vi "Connect to Data Server.vi"(8 "error in (no error)":errorcluster, 9 "timeout ms (60000)":i32=60000, 11 "server address":string) -> (0 "error out":errorcluster, 1 "timed out?":bool, 2 "framework configuration":T1, 3 "server ID":refnum<k5>)   [LabVIEW 2017, in "DSF Core.lvlib"]
uses:
  DSF Core.lvlib
  Typedefs/DSF Engine Framework Configuration.ctl
  Typedefs/DSF Engine Plugin Configuration.ctl
  Typedefs/DSF Timing Info.ctl
  Typedefs/DSF Engine Plugin Thread Configuration.ctl
  Typedefs/DSF Settings Info.ctl
  Typedefs/DSF Engine Transfer Group Configuration.ctl
  Typedefs/DSF Direction.ctl
  Typedefs/DSF Engine Transfer Configuration.ctl
  Typedefs/DSF Byte Order.ctl
  Typedefs/DSF Engine Channel Configuration.ctl
  Typedefs/DSF Data Type.ctl
  Typedefs/DSF Timeout Behavior.ctl
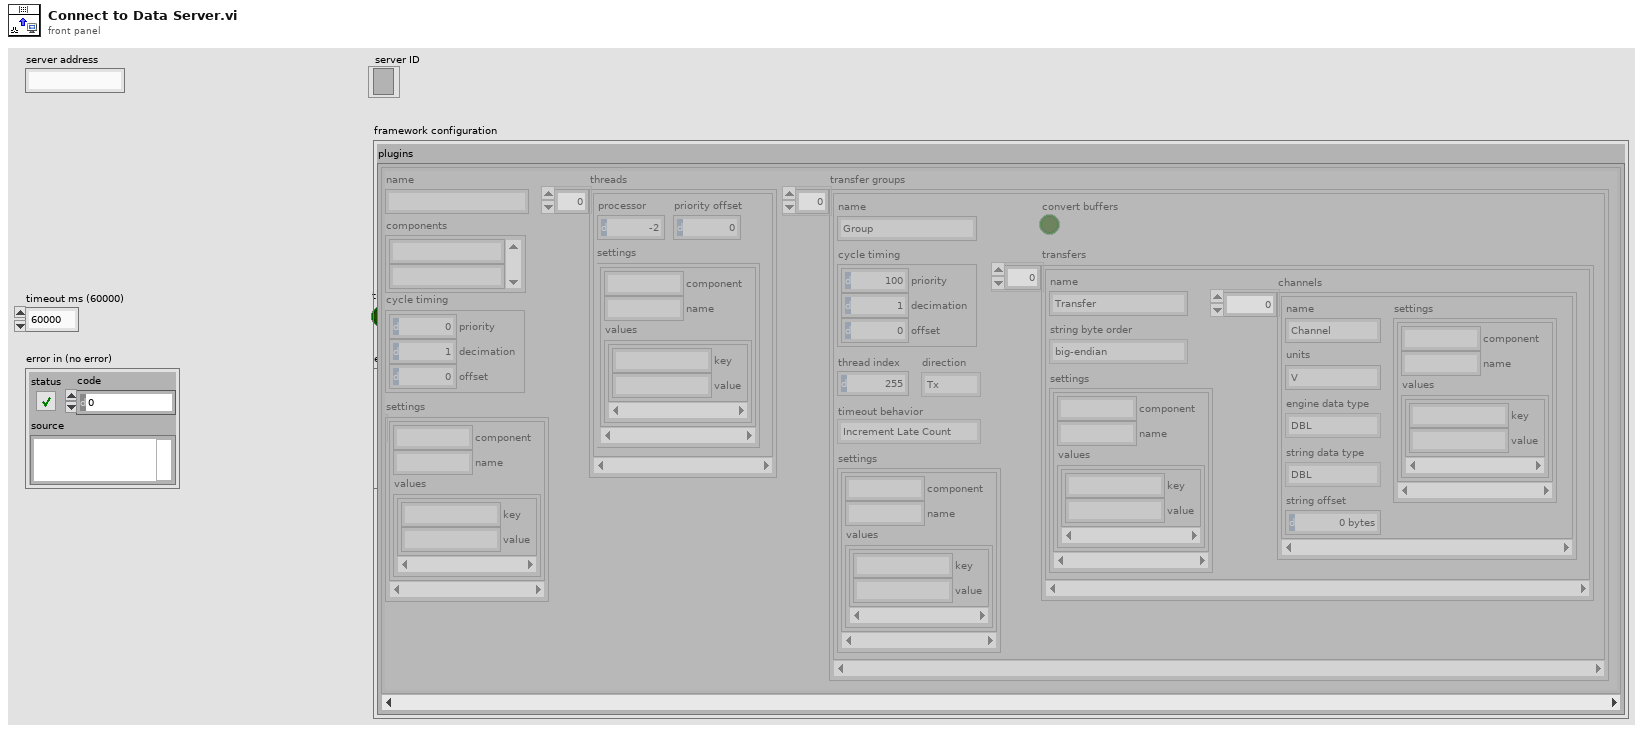
[diagram p1: front panel]
types:
  T1 = typedef "DSF Core.lvlib/DSF Engine Framework Configuration.ctl" = cluster{"plugins":T2[]}
  T2 = typedef "DSF Core.lvlib/DSF Engine Plugin Configuration.ctl" = cluster{"name":string, "components":string[], "cycle timing":T3, "threads":T4[], "transfer groups":T6[], "settings":T5}
  T3 = typedef "DSF Core.lvlib/DSF Timing Info.ctl" = cluster{"priority":u64, "decimation":u64, "offset":u64}
  T4 = typedef "DSF Core.lvlib/DSF Engine Plugin Thread Configuration.ctl" = cluster{"processor":i32, "priority offset":i16, "settings":T5}
  T5 = typedef "DSF Core.lvlib/DSF Settings Info.ctl" = cluster{"component":string, "name":string, "values":cluster{"key":string, "value":string}[]}[]
  T6 = typedef "DSF Core.lvlib/DSF Engine Transfer Group Configuration.ctl" = cluster{"name":string, "direction":T7, "cycle timing":T3, "thread index":u8, "settings":T5, "transfers":T8[], "timeout behavior":T12, "convert buffers":bool}
  T7 = typedef "DSF Core.lvlib/DSF Direction.ctl" = enum8{"Tx", "Rx"}
  T8 = typedef "DSF Core.lvlib/DSF Engine Transfer Configuration.ctl" = cluster{"name":string, "string byte order":T9, "settings":T5, "channels":T10[]}
  T9 = typedef "DSF Core.lvlib/DSF Byte Order.ctl" = enum8{"big-endian", "little-endian"}
  T10 = typedef "DSF Core.lvlib/DSF Engine Channel Configuration.ctl" = cluster{"string offset":u64, "name":string, "units":string, "engine data type":T11, "string data type":T11, "settings":T5}
  T11 = typedef "DSF Core.lvlib/DSF Data Type.ctl" = enum8{"Bool", "SGL", "DBL", "I8", "I16", "I32", "I64", "U8", "U16", "U32", "U64"}
  T12 = typedef "DSF Core.lvlib/DSF Timeout Behavior.ctl" = enum8{"Increment Late Count", "Throw Error"}
  T13 = enum16{"big-endian, network order", "native, host order", "little-endian"}
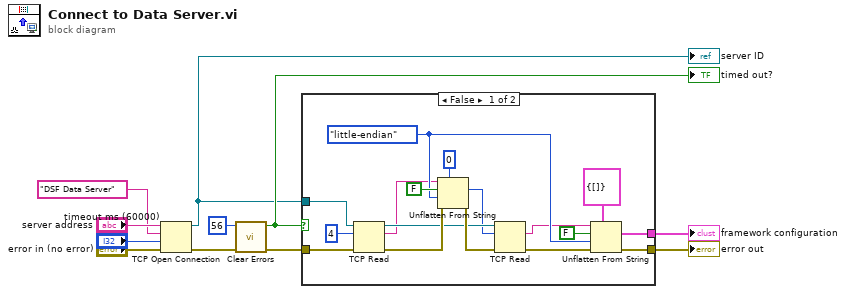
[diagram p0: block diagram]
diagram:
  n1 = TCP Open Connection(address="server address", remote port or service name="DSF Data Server" ("address"), timeout ms (60000)="timeout ms (60000)", error in (no error)="error in (no error)") -> (connection ID=w2:refnum<k5>, error out=w6:errorcluster)  [unwired: 1 in]
  "server ID" <- w2
  n2 = call <vilib>:"Clear Errors.vi"("error in (no error)"=w6, "specific error code to clear (0: all)"=56) -> ("error out"=w5:errorcluster, "specific error cleared?"=w4:bool)  [unwired: 4 in]
  "timed out?" <- w4
  n3 = case shown="False" w4 {
    tunnel: w5 -> [w28 w29]
    tunnel: [w18 w29] -> w3
    tunnel: w2 -> [w27 _]
    tunnel: [w15 _] -> w1
    frame False {
      w16 = T13."little-endian" ("byte order (0:big-endian, network order)")
      n4 = TCP Read(connection ID=w27, bytes to read=4, error in (no error)=w28) -> (connection ID out=w21:refnum<k5>, data out=w14:string, error out=w25:errorcluster)  [unwired: 2 in]
      n5 = Unflatten From String(type=0, binary string=w14, data includes array or string size? (T)=FALSE, byte order (0:big-endian, network order)=w16, error in (no error)=w25) -> (value=w12:i32, error out=w22:errorcluster)  [unwired: 1 out]
      n6 = TCP Read(connection ID=w21, bytes to read=w12, error in (no error)=w22) -> (data out=w13:string, error out=w19:errorcluster)  [unwired: 2 in, 1 out]
      n7 = Unflatten From String(type=T1 {"plugins"=[]} ("Framework Configuration"), binary string=w13, data includes array or string size? (T)=FALSE, byte order (0:big-endian, network order)=w16, error in (no error)=w19) -> (value=w15:T1, error out=w18:errorcluster)  [unwired: 1 out]
    }
    frame True {
    }
  }
  "error out" <- w3
  "framework configuration" <- w1
